vi "H5Fget_obj_ids.vi"(6 "error in (no error)":errorcluster, 8 "Object types":T2=31 items=["H5F_OBJ_FILE"=1, "H5F_OBJ_DATASET"=2, "H5F_OBJ_GROUP"=4, "H5F_OBJ_DATATYPE"=8, "H5F_OBJ_ATTR"=16, "H5F_OBJ_ALL"=31, "H5F_OBJ_LOCAL"=32], 9 "HDF5 File Ref (All open files)":T1) -> (0 "error out":errorcluster, 2 "Object IDs":T1[](array[typedef]), 3 "HDF5 Ref out":T1)   [LabVIEW 2017]
doc: "Returns a list of open object identifiers."
uses:
  <vilib>/UPVI/lvhdf5/library.llb/HDF5 Ref.ctl
  <vilib>/UPVI/lvhdf5/file.llb/H5F_obj_types_t.ctl
  <vilib>/UPVI/lvhdf5/hdf5.dll
panel:
  # "LVHDF5 Toolkit\nCopyright (c) 2005-2013 by Jason D. Sommerville\nCopyright (c) 2014 by UPVI, LLC.\n\nThis use and distribution of this file is governed by the terms found in \nLICENSE.txt distributed with this toolkit and installed at\n <user.lib>\\_lvhdf5\\LICENSE.txt"
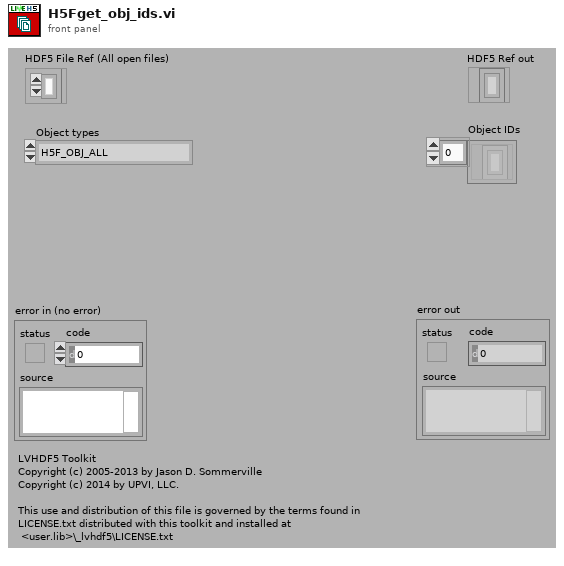
[diagram p1: front panel]
types:
  T1 = typedef "HDF5 Ref.ctl" = refnum<k1>
  T2 = typedef "H5F_obj_types_t.ctl" = u32
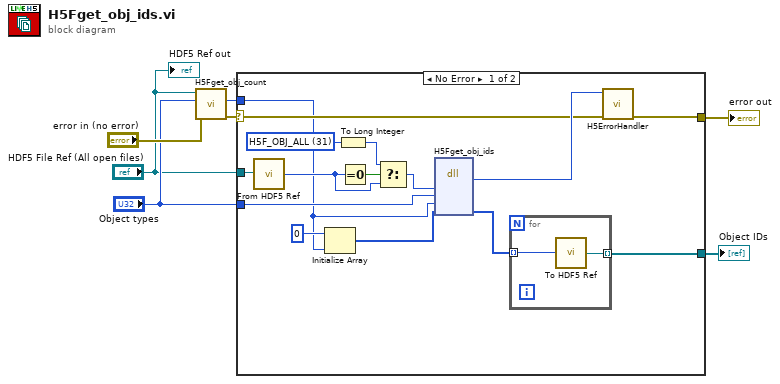
[diagram p0: block diagram]
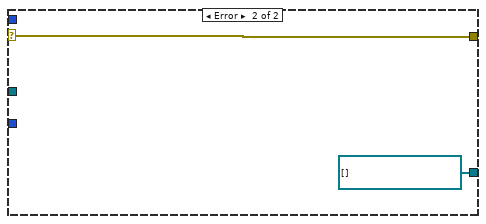
[diagram p2: hidden frame]
diagram:
  n1 = call <vilib>:"H5Fget_obj_count.vi"("Object types"="Object types", "HDF5 File Ref (All open files)"="HDF5 File Ref (All open files)") -> ("Count"=w2:i32)  [unwired: 5 in, 2 out]
  n2 = case shown="No Error" "error in (no error)" {
    selector: "error in (no error)" -> [w18 w25]
    tunnel: [w20 w25] -> w5
    tunnel: "HDF5 File Ref (All open files)" -> [w21 _]
    tunnel: "Object types" -> [w17 _]
    tunnel: w2 -> [w9 _]
    tunnel: [w7 w24] -> w1
    frame No Error {
      w14 = T2 31 items=["H5F_OBJ_FILE"=1, "H5F_OBJ_DATASET"=2, "H5F_OBJ_GROUP"=4, "H5F_OBJ_DATATYPE"=8, "H5F_OBJ_ATTR"=16, "H5F_OBJ_ALL"=31, "H5F_OBJ_LOCAL"=32] ("Object types")
      n3 = call <vilib>:"From HDF5 Ref.vi"("HDF5 Ref"=w21) -> ("I32"=w15:i32)
      n4 = Initialize Array(0, w9) -> (w10:i32[])
      n5 = To Long Integer(number=w14) -> (32bit integer=w12:i32)
      n6 = Equal To 0?(x=w15) -> (x = 0?=w16:bool)
      n7 = Select(t=w12, s=w16, f=w15) -> (s? t:f=w13:i32)
      n8 = dll-call lib="C:/Program Files/National Instruments/LabVIEW 2017/vi.lib/UPVI/lvhdf5/hdf5.dll" fn="H5Fget_obj_ids"("file_id"=w13, "types"=w17, "max_objs"=w9, "obj_id_list"=w10) -> ("return type"=w19:i64, "obj_id_list"=w8:i32[])  [unwired: 6 in, 2 out]
      n9 = for {
        tunnel: w8 -> [w23] mode=indexing
        tunnel: [w22] -> w7 mode=indexing
        n10 = call <vilib>:"To HDF5 Ref.vi"("I32"=w23) -> ("HDF5 Ref"=w22:T1)
      }
      n11 = call <vilib>:"H5ErrorHandler.vi"("error in (no error)"=w18, "herr_t"=w19) -> ("error out"=w20:errorcluster)  [unwired: 3 in, 4 out]
    }
    frame Error {
      w24 = T1[] [] items=["HDF5 Ref"]
    }
  }
  "error out" <- w5
  "Object IDs" <- w1
  "HDF5 Ref out" <- "HDF5 File Ref (All open files)"
